vi "Facade Donut Chart.vi"(0 "Data In":T4, 2 "Display State In":T2, 3 "Container State":T3) -> (6 "Data Out":T4, 7 "Display State Out":T2, 8 "Action":T1)   [LabVIEW 2020, in "Donut Chart.xctl"]
uses:
  Donut Chart.xctl
  Data Donut Chart.ctl
  <vilib>/_xctls/Container State.ctl
  State Donut Chart.ctl
  <vilib>/_xctls/Action.ctl
  <vilib>/_xctls/XControlSupport.lvlib
panel:
  in  "ActiveX Container":refnum<k7>(container)
types:
  T1 = typedef "XControlSupport.lvlib/Action.ctl" = cluster{"Data Changed?":bool, "State Changed?":bool, "Action Name":string}
  T2 = typedef "Donut Chart.xctl/State Donut Chart.ctl" = cluster{"Numeric":dbl}
  T3 = typedef "XControlSupport.lvlib/Container State.ctl" = cluster{"Indicator?":bool, "Run Mode?":bool, " Refnum":refnum<vi>}
  T4 = typedef "Donut Chart.xctl/Data Donut Chart.ctl" = cluster{"Plot Title":string, "Plots":cluster{"Name":string, "Value":dbl, "Color":u32}[]}
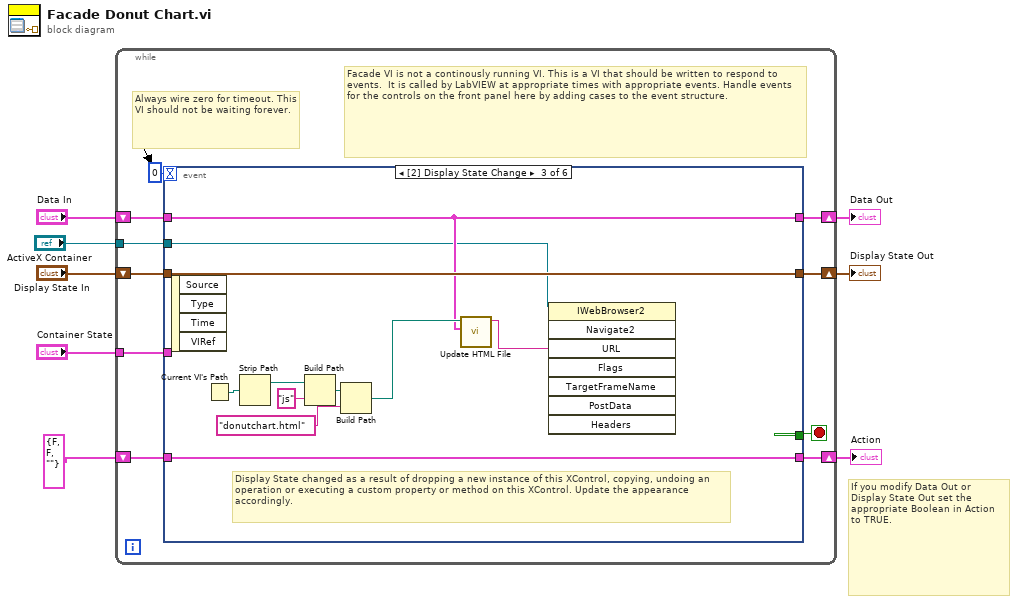
[diagram p0: block diagram]
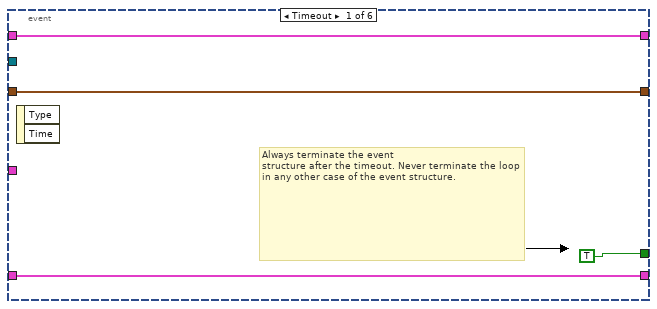
[diagram p2: hidden frame]
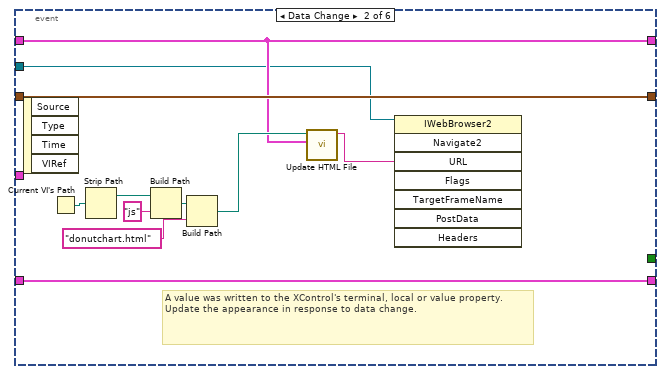
[diagram p3: hidden frame]
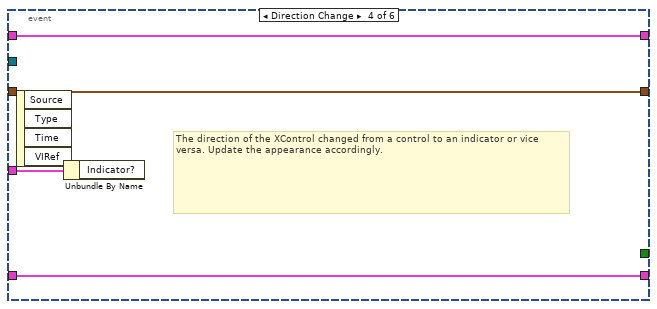
[diagram p4: hidden frame]
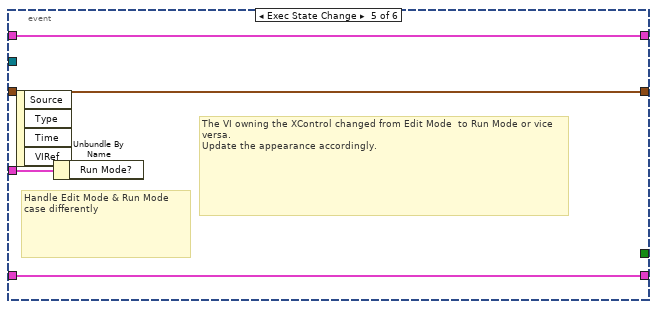
[diagram p5: hidden frame]
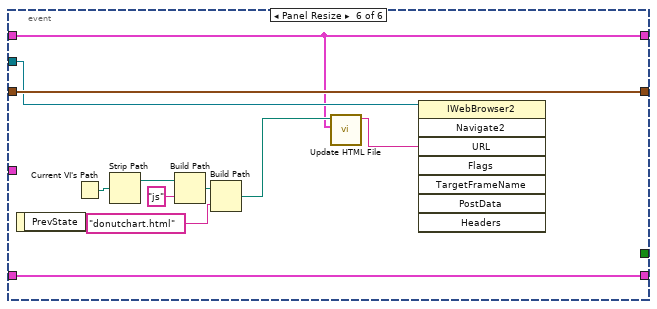
[diagram p6: hidden frame]
diagram:
  # "If you modify Data Out or\nDisplay State Out set the\nappropriate Boolean in Action\nto TRUE."
  n1 = while {
    shift-right: [w17] -> w5
    shift-left: "Display State In" -> [w18]
    tunnel: "Container State" -> [w14]
    shift-right: [w12] -> w8
    shift-left: "Data In" -> [w13]
    shift-right: [w10] -> w3
    shift-left: T1 {"Data Changed?"=FALSE, "State Changed?"=FALSE, "Action Name"=""} ("Action") -> [w11]
    tunnel: "ActiveX Container" -> [w9]
    stop <- w16 stop-if-true
    # "Facade VI is not a continously running VI. This is a VI that should be written to respond to events.  It is called by LabVIEW at appropriate times with appropriate events. Handle events for the controls on the front panel here by adding cases to the event structure."
    # "Always wire zero for timeout. This\nVI should not be waiting forever."
    n2 = event shown="[2] Display State Change" {
      selector: _ -> [_ _ _ _ _ _]
      dyn-events: _ -> [_ _ _ _ _ _]
      timeout: 0 -> [_ _ _ _ _ _]
      tunnel: w18 -> [w20 w33 w44 w47 w51 w63]
      tunnel: [w20 w33 w44 w47 w51 w63] -> w17
      tunnel: [TRUE _ _ _ _ _] -> w16
      tunnel: w14 -> [_ _ _ w48 w52 _]
      tunnel: w13 -> [w19 w25 w35 w46 w50 w53]
      tunnel: [w19 w25 w35 w46 w50 w53] -> w12
      tunnel: [w21 w32 w43 w45 w49 w62] -> w10
      tunnel: w11 -> [w21 w32 w43 w45 w49 w62]
      tunnel: w9 -> [_ w24 w34 _ _ w54]
      event Timeout {
        # "Always terminate the event\nstructure after the timeout. Never terminate the loop in any other case of the event structure."
        n3 = event-data() -> ()  [unwired: 1 in, 2 out]
      }
      event Data Change {
        # "A value was written to the XControl's terminal, local or value property.\nUpdate the appearance in response to data change."
        n4 = event-data() -> ()  [unwired: 1 in, 4 out]
        n5 = Current VI's Path() -> (path=w31:path)
        n6 = Strip Path(path=w31) -> (stripped path=w30:path)  [unwired: 1 out]
        n7 = Build Path(base path=w30, name or relative path="js") -> (appended path=w28:path)
        n8 = Build Path(base path=w28, name or relative path="donutchart.html") -> (appended path=w26:path)
        n9 = call "Update HTML File.vi"("Plot Data"=w25, "Path"=w26) -> ("URL out"=w23:string)  [unwired: 9 in]
        n10 = invoke class="IWebBrowser2" method="Navigate2"(reference=w24, "URL"=w23) -> ()  [unwired: 6 in, 8 out]
      }
      event Display State Change {
        # "Display State changed as a result of dropping a new instance of this XControl, copying, undoing an operation or executing a custom property or method on this XControl. Update the appearance accordingly."
        n11 = event-data() -> ()  [unwired: 1 in, 4 out]
        n12 = Current VI's Path() -> (path=w42:path)
        n13 = Strip Path(path=w42) -> (stripped path=w41:path)  [unwired: 1 out]
        n14 = Build Path(base path=w41, name or relative path="js") -> (appended path=w39:path)
        n15 = Build Path(base path=w39, name or relative path="donutchart.html") -> (appended path=w37:path)
        n16 = call "Update HTML File.vi"("Plot Data"=w35, "Path"=w37) -> ("URL out"=w36:string)  [unwired: 9 in]
        n17 = invoke class="IWebBrowser2" method="Navigate2"(reference=w34, "URL"=w36) -> ()  [unwired: 6 in, 8 out]
      }
      event Direction Change {
        # "The direction of the XControl changed from a control to an indicator or vice versa. Update the appearance accordingly."
        n18 = event-data() -> ()  [unwired: 1 in, 4 out]
        n19 = Unbundle By Name(w48) -> ()  [unwired: 1 out]
      }
      event Exec State Change {
        # "The VI owning the XControl changed from Edit Mode  to Run Mode or vice versa.\nUpdate the appearance accordingly."
        # "Handle Edit Mode & Run Mode\ncase differently"
        n20 = event-data() -> ()  [unwired: 1 in, 4 out]
        n21 = Unbundle By Name(w52) -> ()  [unwired: 1 out]
      }
      event Panel Resize {
        n22 = event-data() -> ()  [unwired: 1 in, 1 out]
        n23 = Current VI's Path() -> (path=w61:path)
        n24 = Strip Path(path=w61) -> (stripped path=w60:path)  [unwired: 1 out]
        n25 = Build Path(base path=w60, name or relative path="js") -> (appended path=w58:path)
        n26 = Build Path(base path=w58, name or relative path="donutchart.html") -> (appended path=w56:path)
        n27 = call "Update HTML File.vi"("Plot Data"=w53, "Path"=w56) -> ("URL out"=w55:string)  [unwired: 9 in]
        n28 = invoke class="IWebBrowser2" method="Navigate2"(reference=w54, "URL"=w55) -> ()  [unwired: 6 in, 8 out]
      }
    }
  }
  "Display State Out" <- w5
  "Data Out" <- w8
  "Action" <- w3
